vi "LakeShore Ramp Act.vi"(0 "command text in":string[](array[string])) -> ()   [LabVIEW 2020]
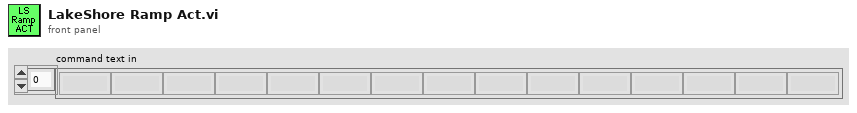
[diagram p1: front panel]
types:
  T1 = typedef "LSRamp.ctl" = cluster{"VISA Resource Name":refnum<visa-resource-name>, "extra wait":i32, "start (K/W)":dbl, "end (K/W)":dbl, "Sweep Time (H:M:S)":dbl, "Mapping":bool, "Parameter":bool, "Loop":bool}
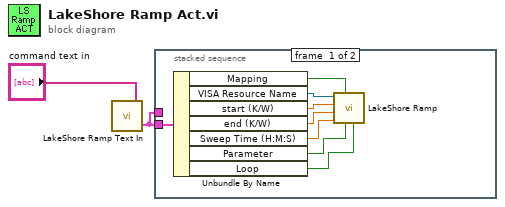
[diagram p0: block diagram]
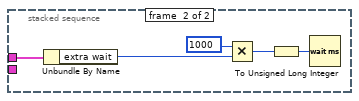
[diagram p2: hidden frame]
diagram:
  n1 = call "LakeShore Ramp Text In.vi"("command text in"="command text in") -> ("LSRamp"=w1:T1)  [unwired: 4 in]
  n2 = stacked-sequence {
    tunnel: w1 -> [w10 _]
    tunnel: w1 -> [_ w12]
    frame #0 {
      n3 = Unbundle By Name(w10) -> ("Mapping"=w9:bool, "VISA Resource Name"=w8:refnum<visa-resource-name>, "start (K/W)"=w7:dbl, "end (K/W)"=w6:dbl, "Sweep Time (H:M:S)"=w5:dbl, "Parameter"=w4:bool, "Loop"=w3:bool)
      n4 = call "LakeShore Ramp.vi"("Loop"=w3, "Parameter"=w4, "Mapping"=w9, "Time (Hr:Min:Sec)"=w5, "End Temp/Power"=w6, "Start Temp/Power"=w7, "VISA resource name"=w8) -> ()  [unwired: 5 in]
    }
    frame #1 {
      n5 = Unbundle By Name(w12) -> ("extra wait"=w11:i32)
      n6 = Multiply(x=1000 ("y"), y=w11) -> (x*y=w14:i32)
      n7 = To Unsigned Long Integer(number=w14) -> (unsigned 32bit integer=w13:u32)
      n8 = Wait (ms)(milliseconds to wait=w13) -> ()  [unwired: 1 out]
    }
  }
